vi "Periodic Tasks.vi"(8 "error in":errorcluster) -> ()   [LabVIEW 2016]
doc: "This VI runs in parallel to other tasks. It can contain as many user-defined periodic loops as you need. These can carry out PID or other sorts of timed response."
uses:
  <vilib>/Rock Robotics/WPI/Solenoid/WPI_SolenoidValue.ctl
  <vilib>/Rock Robotics/WPI/Utilities/WPI_GetSetVariantRefNum.vi
  Robot Global Data.vi
  <vilib>/Rock Robotics/WPI/Solenoid/WPI_SolenoidSetEnum.vi
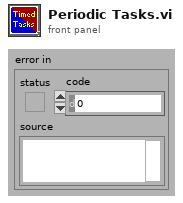
[diagram p1: front panel]
types:
  T1 = typedef "WPI_JoystickDevRef.ctl" = cluster{"Device":T2}
  T2 = typedef "WPI_JoystickDeviceEnum.ctl" = enum16{"USB 0", "USB 1", "USB 2", "USB 3", "USB 4", "USB 5"}
  T3 = typedef "WPI_RobotDriveDevRef.ctl" = cluster{"DevStatus":errorcluster, "Motors[]":T4[], "Square Inputs":bool, "Max Output":dbl}
  T4 = typedef "WPI_MotorControlDeviceRef.ctl" = cluster{"DeviceStatus":errorcluster, "Type":T5, "PWM":cluster{"PWM Channel":T6, "DeadBand":T7}, "CAN":cluster{"Device Number":u8, "SetOutput VI Ref":variant, "GetOutput VI Ref":variant, "Enable VI Ref":variant, "Disable VI Ref":variant, "Data":variant}, "Invert":bool}
  T5 = typedef "WPI_MotorControlType.ctl" = enum16{"PWM", "CAN"}
  T6 = typedef "FPGA_DIOPWMChannel.ctl" = enum8{"PWM 0", "PWM 1", "PWM 2", "PWM 3", "PWM 4", "PWM 5", "PWM 6", "PWM 7", "PWM 8", "PWM 9", "PWM MXP 0", "PWM MXP 1", "PWM MXP 2", "PWM MXP 3", "PWM MXP 4", "PWM MXP 5", "PWM MXP 6", "PWM MXP 7", "PWM MXP 8", "PWM MXP 9", "Invalid"}
  T7 = typedef "WPI_PWMDeadband.ctl" = cluster{"Name":string, "maxPositivePwm":i32, "minPositivePwm":i32, "centerPwm":i32, "maxNegativePwm":i32, "minNegativePwm":i32, "angularRange":u16}
  T8 = cluster{"JoystickDevRef":T1, "RobotDriveDevRef":T3}
  T9 = typedef "WPI_DigitalInputDevRef.ctl" = cluster{"DevStatus":errorcluster, "DIO Channel":T10}
  T10 = typedef "FPGA_DIOChannel.ctl" = enum8{"DIO 0", "DIO 1", "DIO 2", "DIO 3", "DIO 4", "DIO 5", "DIO 6", "DIO 7", "DIO 8", "DIO 9", "DIO MXP 0", "DIO MXP 1", "DIO MXP 2", "DIO MXP 3", "DIO MXP 4", "DIO MXP 5", "DIO MXP 6", "DIO MXP 7", "DIO MXP 8", "DIO MXP 9", "DIO MXP 10", "DIO MXP 11", "DIO MXP 12", "DIO MXP 13", "DIO MXP 14", "DIO MXP 15", "SPI Port CS1", "SPI Port CS2", "SPI Port CS3", "SPI Port MISO", "SPI Port MOSI", "Invalid"}
  T11 = typedef "WPI_SolenoidValue.ctl" = enum16{"Off", "On", "Forward", "Reverse"}
  T12 = typedef "WPI_SolenoidDevRef.ctl" = cluster{"DevStatus":errorcluster, "Pneumatics Control Module":u8, "Forward Solenoid Channel":T13, "Reverse Solenoid Channel":T13}
  T13 = typedef "WPI_SolenoidChannel.ctl" = enum8{"Solenoid 0", "Solenoid 1", "Solenoid 2", "Solenoid 3", "Solenoid 4", "Solenoid 5", "Solenoid 6", "Solenoid 7", "Invalid"}
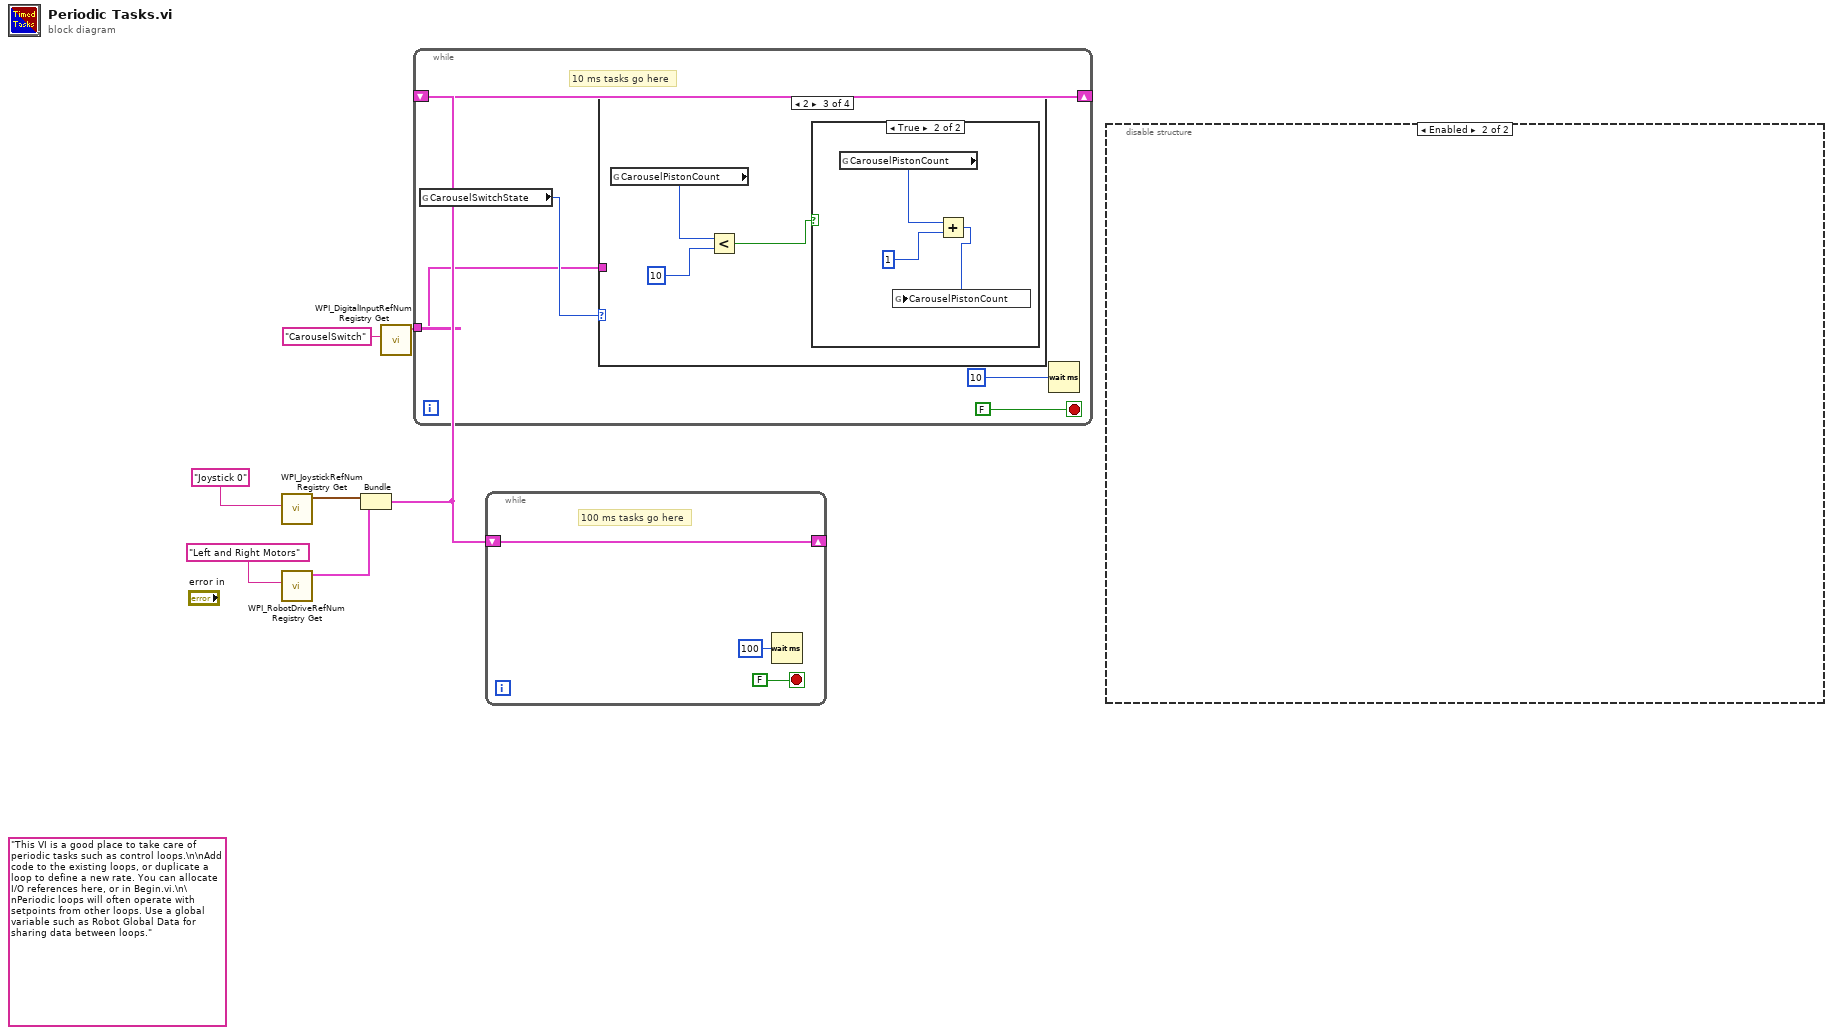
[diagram p0: block diagram]
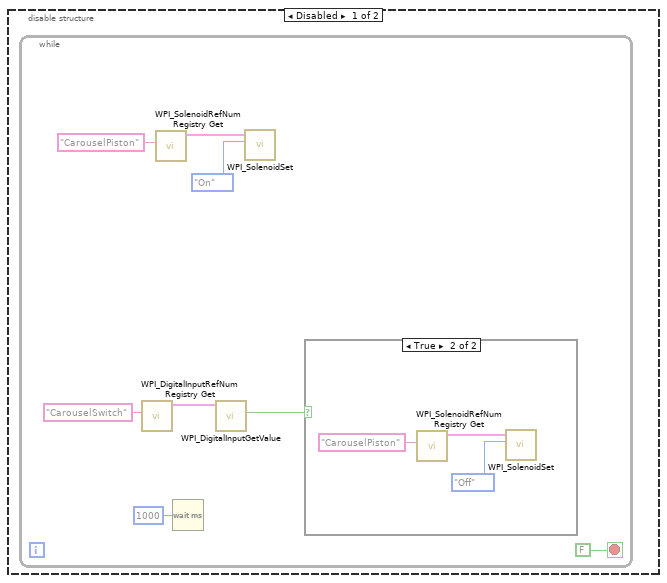
[diagram p2: hidden frame]
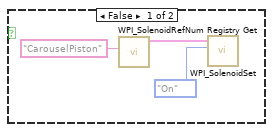
[diagram p3: hidden frame]
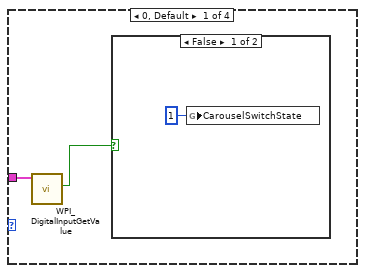
[diagram p4: hidden frame]
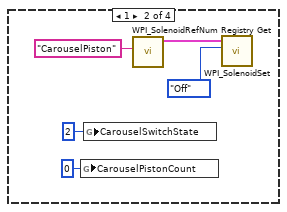
[diagram p6: hidden frame]
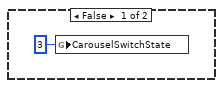
[diagram p7: hidden frame]
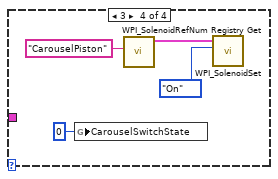
[diagram p8: hidden frame]
diagram:
  (unwired) "This VI is a good place to take care of periodic tasks such as control loops.\n\nAdd code to the existing loops, or duplicate a loop to define a new rate. You can allocate I/O references here, or in Begin.vi.\n\nPeriodic loops will often operate with setpoints from other loops. Use a global variable such as Robot Global Data for sharing data between loops."
  n1 = call <vilib>:"WPI_JoystickRefNum Registry Get.vi"("refnum name"="Joystick 0") -> ("JoystickDevRef"=w5:T1)  [unwired: 1 in, 9 out]
  n2 = call <vilib>:"WPI_RobotDriveRefNum Registry Get.vi"("refnum name"="Left and Right Motors") -> ("RobotDriveDevRef"=w4:T3)  [unwired: 1 in, 9 out]
  n3 = Bundle("JoystickDevRef"=w5, "RobotDriveDevRef"=w4) -> (w3:T8)  [unwired: 1 out]
  n4 = call <vilib>:"WPI_DigitalInputRefNum Registry Get.vi"("refnum name"="CarouselSwitch") -> ("DigitalInputDevRef"=w1:T9)  [unwired: 9 in, 1 out]
  n5 = while {
    shift-right: [w10] -> _
    shift-left: w3 -> [w10]
    tunnel: w1 -> [w8]
    stop <- FALSE stop-if-true
    # "10 ms tasks go here"
    n6 = global read "Robot Global Data.vi" "CarouselSwitchState"() -> (w9:u8)
    n7 = case shown="2" w9 {
      tunnel: w8 -> [w14 _ _ _]
      frame 0, Default {
        n8 = call <vilib>:"WPI_DigitalInputGetValue.vi"("DigitalInputDevRef"=w14) -> ("Value"=w13:bool)  [unwired: 8 in, 2 out]
        n9 = case shown="False" w13 {
          frame False {
            n10 = global write "Robot Global Data.vi" "CarouselSwitchState"(u8 1 ("CarouselSwitchState")) -> ()
          }
          frame True {
          }
        }
      }
      frame 1 {
        n11 = global write "Robot Global Data.vi" "CarouselPistonCount"(u8 0 ("CarouselSwitchState")) -> ()
        n12 = global write "Robot Global Data.vi" "CarouselSwitchState"(u8 2 ("CarouselSwitchState")) -> ()
        n13 = call <vilib>:"WPI_SolenoidRefNum Registry Get.vi"("refnum name"="CarouselPiston") -> ("SolenoidDevRef"=w19:T12)  [unwired: 9 in, 1 out]
        n14 = call-poly <vilib>:"WPI_SolenoidSet.vi"("Value"=WPI_SolenoidValue."Off", "SolenoidDevRef"=w19) -> ()  [unwired: 8 in, 2 out]
      }
      frame 2 {
        n15 = global read "Robot Global Data.vi" "CarouselPistonCount"() -> (w23:u8)
        n16 = Less?(x=w23, y=u8 10) -> (x < y?=w21:bool)
        n17 = case shown="True" w21 {
          frame False {
            n18 = global write "Robot Global Data.vi" "CarouselSwitchState"(u8 3 ("CarouselSwitchState")) -> ()
          }
          frame True {
            n19 = global read "Robot Global Data.vi" "CarouselPistonCount"() -> (w27:u8)
            n20 = Add(x=w27, y=u8 1) -> (x+y=w25:u8)
            n21 = global write "Robot Global Data.vi" "CarouselPistonCount"(w25) -> ()
          }
        }
      }
      frame 3 {
        n22 = global write "Robot Global Data.vi" "CarouselSwitchState"(u8 0 ("CarouselSwitchState")) -> ()
        n23 = call <vilib>:"WPI_SolenoidRefNum Registry Get.vi"("refnum name"="CarouselPiston") -> ("SolenoidDevRef"=w30:T12)  [unwired: 9 in, 1 out]
        n24 = call-poly <vilib>:"WPI_SolenoidSet.vi"("Value"=WPI_SolenoidValue."On", "SolenoidDevRef"=w30) -> ()  [unwired: 8 in, 2 out]
      }
    }
    n25 = Wait (ms)(milliseconds to wait=u32 10) -> ()  [unwired: 1 out]
  }
  n26 = while {
    shift-right: [w32] -> _
    shift-left: w3 -> [w32]
    stop <- FALSE stop-if-true
    # "100 ms tasks go here"
    n27 = Wait (ms)(milliseconds to wait=u32 100) -> ()  [unwired: 1 out]
  }
  n28 = disable-structure shown="Enabled" {
    frame Disabled {
      n29 = while {
        stop <- FALSE stop-if-true
        n30 = call <vilib>:"WPI_DigitalInputRefNum Registry Get.vi"("refnum name"="CarouselSwitch") -> ("DigitalInputDevRef"=w37:T9)  [unwired: 9 in, 1 out]
        n31 = call <vilib>:"WPI_SolenoidRefNum Registry Get.vi"("refnum name"="CarouselPiston") -> ("SolenoidDevRef"=w40:T12)  [unwired: 9 in, 1 out]
        n32 = Wait (ms)(milliseconds to wait=u32 1000) -> ()  [unwired: 1 out]
        n33 = call <vilib>:"WPI_DigitalInputGetValue.vi"("DigitalInputDevRef"=w37) -> ("Value"=w36:bool)  [unwired: 8 in, 2 out]
        n34 = call-poly <vilib>:"WPI_SolenoidSet.vi"("Value"=WPI_SolenoidValue."On", "SolenoidDevRef"=w40) -> ()  [unwired: 8 in, 2 out]
        n35 = case shown="True" w36 {
          frame False {
            n36 = call <vilib>:"WPI_SolenoidRefNum Registry Get.vi"("refnum name"="CarouselPiston") -> ("SolenoidDevRef"=w44:T12)  [unwired: 9 in, 1 out]
            n37 = call-poly <vilib>:"WPI_SolenoidSet.vi"("Value"=WPI_SolenoidValue."On", "SolenoidDevRef"=w44) -> ()  [unwired: 8 in, 2 out]
          }
          frame True {
            n38 = call <vilib>:"WPI_SolenoidRefNum Registry Get.vi"("refnum name"="CarouselPiston") -> ("SolenoidDevRef"=w47:T12)  [unwired: 9 in, 1 out]
            n39 = call-poly <vilib>:"WPI_SolenoidSet.vi"("Value"=WPI_SolenoidValue."Off", "SolenoidDevRef"=w47) -> ()  [unwired: 8 in, 2 out]
          }
        }
      }
    }
    frame Enabled {
    }
  }
